vi "intensity average and center.vi"() -> ()   [LabVIEW 2011]
uses:
  <vilib>/Analysis/NI_AALBase.lvlib
panel:
  out "error":i32
  out "mean":dbl format="%0.2f"
  out "Array":dbl[](array[numeric])
  in  "N loops":i32
  in  "Time Target (s)":dbl=10.0
  in  "rate (Hz)":dbl=100.0 format="%0.2f"
  in  "Y pos":dbl=35.0
  in  "X Pos":dbl=192.0
  in  "Y Parameters":T1={"Number of Y Steps"=200, "Max Y (V)"=2.0, "Min Y (V)"=-2.0}
  in  "X Parameters":T2={"Number of X Steps"=200, "Max X (V)"=2.0, "Min X (V)"=-2.0}
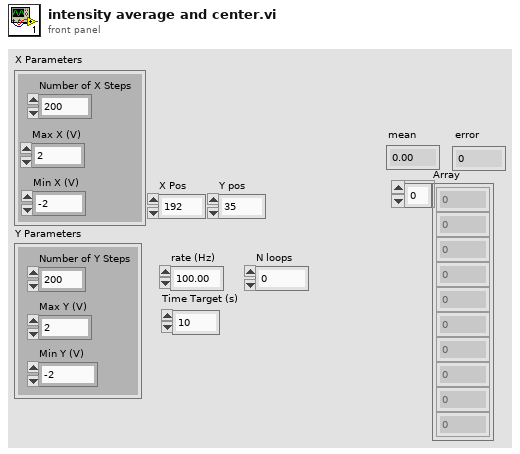
[diagram p1: front panel]
types:
  T1 = cluster{"Number of Y Steps":i32, "Max Y (V)":dbl, "Min Y (V)":dbl}
  T2 = cluster{"Number of X Steps":i32, "Max X (V)":dbl, "Min X (V)":dbl}
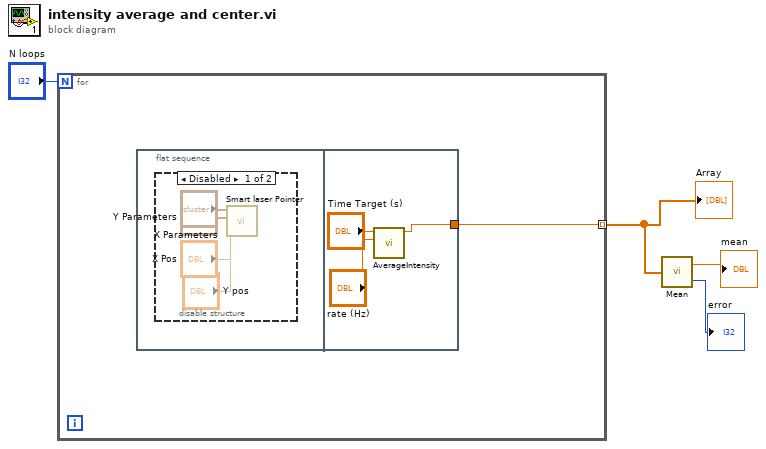
[diagram p0: block diagram]
diagram:
  n1 = for {
    N: "N loops" -> [_]
    tunnel: [w5] -> w3 mode=indexing
    n2 = flat-sequence {
      tunnel: [w10] -> w5
      frame #0 {
        n3 = disable-structure shown="Disabled" {
          frame Disabled {
            n4 = call "Smart laser Pointer.vi"("Y pos"="Y pos", "X Pos"="X Pos", "Y Parameters"="Y Parameters", "X Parameters"="X Parameters") -> ()  [unwired: 8 in]
          }
          frame Enabled {
          }
        }
      }
      frame #1 {
        n5 = call "AverageIntensity.vi"("rate (Hz)"="rate (Hz)", "Time Target (s)"="Time Target (s)") -> ("Average intensity (cts/s)"=w10:dbl)  [unwired: 9 in]
      }
    }
  }
  "Array" <- w3
  n6 = call <vilib>:"Mean.vi"("X"=w3) -> ("mean"=→"mean":dbl, "error"=→"error":i32)
